vi "Control Mode Write Array.vi"(8 "error in":errorcluster, 10 "Control Mode STS":u16[](array[numeric]), 11 "Cycler in":refnum<class "Cycler.lvclass">) -> (0 "error out":errorcluster, 3 "Cycler out":refnum<class "Cycler.lvclass">)   [LabVIEW 2023, in "Cycler.lvclass"]
uses:
  Cycler.lvclass
  Cycler.lvclass/Cycler.ctl
  Low Level Capabilities/Control Mode/Control Mode.lvclass
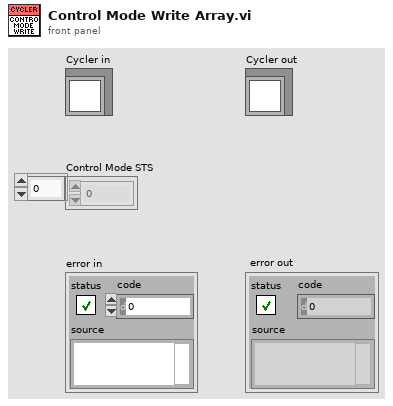
[diagram p1: front panel]
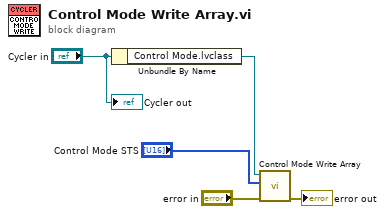
[diagram p0: block diagram]
diagram:
  n1 = Unbundle By Name("Cycler in") -> ("Control Mode.lvclass"=w2:refnum<class "Control Mode.lvclass">)
  n2 = call-dynamic "Control Mode Write Array.vi"("error in"="error in", "Control Mode STS"="Control Mode STS", "Control Mode in"=w2) -> ("error out"=→"error out":errorcluster)  [unwired: 7 in, 1 out]
  "Cycler out" <- "Cycler in"
